vi "tdms.make_channel_name.vi"(8 "error in":errorcluster, 10 "Channel Name":string, 11 "Group Name":string) -> (0 "error out":errorcluster, 3 "channel name":string)   [LabVIEW 2020, in "Nominal Client.lvclass"]
uses:
  Nominal Client.lvclass
  Nominal Client.lvclass/Nominal Client.ctl
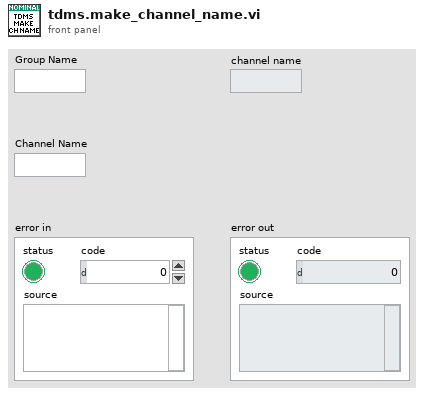
[diagram p1: front panel]
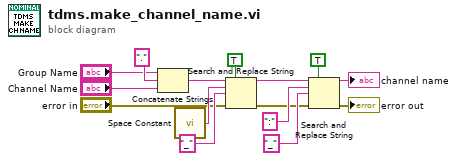
[diagram p0: block diagram]
diagram:
  n1 = Concatenate Strings("Group Name", "." ("string"), "Channel Name") -> (w11:string)
  n2 = call <vilib>:"Space Constant.vi"() -> ("String"=w14:string)
  n3 = Search and Replace String(replace all?=TRUE ("replace all? (F)"), input string=w11, search string=w14, replace string="_", error in="error in") -> (result string=w7:string, error out=w3:errorcluster)  [unwired: 3 in, 2 out]
  n4 = Search and Replace String(replace all?=TRUE ("replace all? (F)"), input string=w7, search string=":", replace string="_", error in=w3) -> (result string=→"channel name":string, error out=→"error out":errorcluster)  [unwired: 3 in, 2 out]
